vi "DAQmx多通道单点输出D.vi"() -> ()   [LabVIEW 2010]
uses:
  <vilib>/DAQmx/write.llb/DAQmx Write.vi
  <vilib>/DAQmx/write.llb/DAQmx Write (Analog 1D DBL NChan 1Samp).vi
  <vilib>/daqmx/miscellaneous.llb/DAQmx Fill In Error Info.vi
panel:
  in  "data":dbl[](array[numeric]) format="%0.2f"
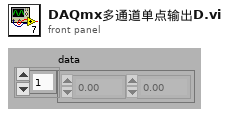
[diagram p1: front panel]
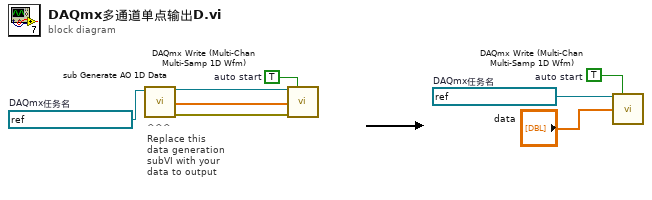
[diagram p0: block diagram]
diagram:
  w3 = TRUE  # auto start
  w2 = refnum<k21> "MyVoltageOutTask"  # DAQmx任务名
  w8 = TRUE  # auto start
  w4 = refnum<k21> "MyVoltageOutTask"  # DAQmx任务名
  # "^^^\nReplace this\ndata generation\nsubVI with your\ndata to output"
  n1 = call <vilib>:"sub Generate AO 1D Data.vi"("task in"=w4) -> ("error out"=w5:errorcluster, "Data"=w6:dbl[], "task out"=w7:refnum<k21>)  [unwired: 8 in]
  n2 = call-poly "DAQmx Write (Multi-Chan Multi-Samp 1D Wfm).vi"("task/channels in"=w7, "auto start"=w8, "data"=w6, "error in"=w5) -> ()  [unwired: 9 in, 3 out]
  n3 = call-poly "DAQmx Write (Multi-Chan Multi-Samp 1D Wfm).vi"("task/channels in"=w2, "auto start"=w3, "data"="data") -> ()  [unwired: 10 in, 3 out]
